vi "Calc Eval.vi"(8 "error in (no error)":errorcluster, 10 "Inputs":dbl[](array[numeric]), 11 "Tare Calc in":refnum<class "Tare Calc.lvclass">) -> (0 "error out":errorcluster, 1 "Additional Updates":T1[](array[typedef]), 2 "Result":dbl, 3 "Tare Calc out":refnum<class "Tare Calc.lvclass">)   [LabVIEW 2020, in "VolatusCalcs.lvlib" / "Tare Calc.lvclass"]
uses:
  Tare Calc.lvclass
  Tare Calc.lvclass/Tare Calc.ctl
  <vilib>/Analysis/NI_AALBase.lvlib
  <vilib>/Analysis/baseanly.llb/Mean (DBL).vi
  Calculation/Additional Update.ctl
  Calculation/Calculation.lvclass
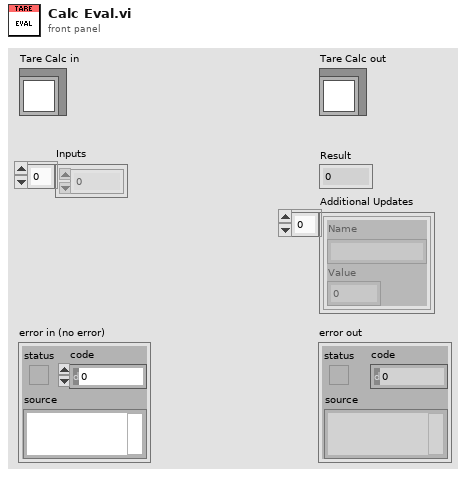
[diagram p1: front panel]
types:
  T1 = typedef "VolatusCalcs.lvlib/Calculation.lvclass/Additional Update.ctl" = cluster{"Name":string, "Value":dbl}
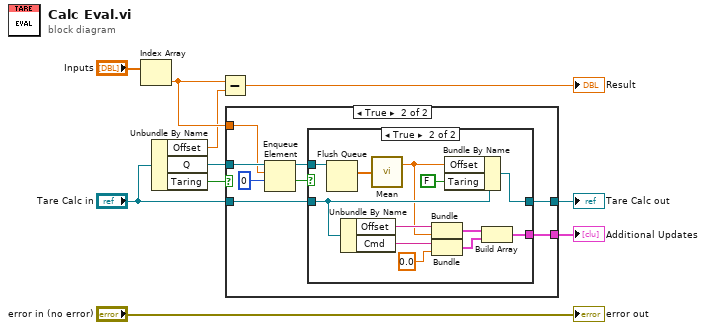
[diagram p0: block diagram]
diagram:
  n1 = Index Array(array="Inputs") -> (element=w5:dbl)  [unwired: 1 in]
  n2 = Unbundle By Name("Tare Calc in") -> ("Offset"=w2:dbl, "Q"=w6:refnum<queue>, "Taring"=w7:bool)
  n3 = Subtract(x=w5, y=w2) -> (x-y=→"Result":dbl)
  n4 = case shown="True" w7 {
    tunnel: w6 -> [_ w19]
    tunnel: w5 -> [_ w18]
    tunnel: "Tare Calc in" -> [w11 w15]
    tunnel: [w11 w13] -> w3
    tunnel: [_ w12] -> w1
    frame False {
    }
    frame True {
      n5 = Enqueue Element(queue=w19, element=w18, timeout in ms (-1)=0) -> (queue out=w14:refnum<queue>, timed out?=w16:bool)  [unwired: 1 in, 1 out]
      n6 = case shown="True" w16 {
        tunnel: w15 -> [w20 w28]
        tunnel: w14 -> [_ w32]
        tunnel: [w20 w29] -> w13
        tunnel: [_ w21] -> w12
        frame False {
        }
        frame True {
          n7 = Flush Queue(queue=w32) -> (remaining elements=w31:dbl[])  [unwired: 1 in, 2 out]
          n8 = Unbundle By Name(w28) -> ("Offset"=w27:string, "Cmd"=w25:string)
          n9 = call-poly <vilib>:"Mean.vi"("X"=w31) -> ("mean"=w26:dbl)  [unwired: 1 out]
          n10 = Bundle("Offset"=w27, "mean"=w26) -> (w23:cluster{"Offset":string, "mean":dbl})  [unwired: 1 in]
          n11 = Bundle("Cmd"=w25, 0.0) -> (w22:cluster{"Cmd":string, dbl})  [unwired: 1 in]
          n12 = Bundle By Name(cluster=w28, "Offset"=w26, "Taring"=FALSE) -> (w29:refnum<class "Tare Calc.lvclass">)
          n13 = Build Array(w23, w22) -> (w21:cluster{"Cmd":string, "mean":dbl}[])
        }
      }
    }
  }
  "Tare Calc out" <- w3
  "Additional Updates" <- w1
  "error out" <- "error in (no error)"
